vi "Handshake.vi"(8 "error in (no error)":errorcluster, 9 "Timeout (5000ms)":i32=5000, 11 "dotNET SSL Socket in":refnum<class "dotNET SSL Server.lvclass">) -> (0 "error out":errorcluster, 3 "dotNET SSL Socket out":refnum<class "dotNET SSL Server.lvclass">)   [LabVIEW 2013, in "dotNET SSL Socket.lvlib" / "dotNET SSL Server.lvclass"]
doc: "Performs the SSL Server handshake."
uses:
  dotNET SSL Server.lvclass
  dotNET SSL Socket/dotNET SSL Socket.lvclass/dotNET SSL Socket.ctl
  dotNET SSL Server.lvclass/dotNET SSL Server.ctl
  dotNET SSL Socket/Read SSLStream.vi
  Read Client Cert Required.vi
  dotNET SSL Socket/Read Check Revocation.vi
  Read Server Certificate.vi
  dotNET SSL Socket/Read Masked SSL Protocols.vi
  dotNET SSL Socket/dotNET SSL Socket.lvclass
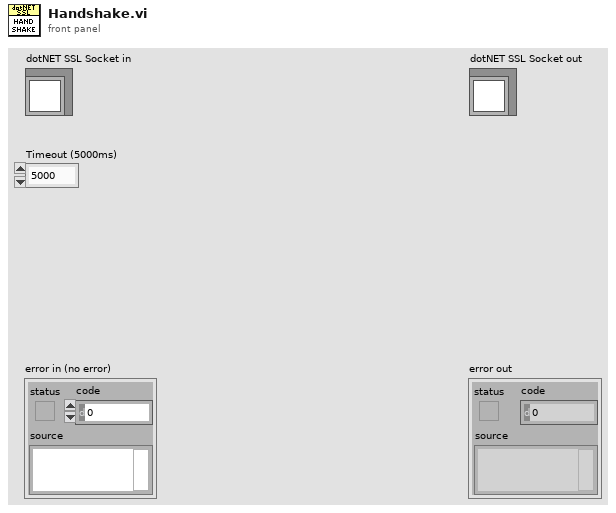
[diagram p1: front panel]
types:
  T1 = typedef "dotNET SSL Socket.lvlib/dotNET SSL Socket.lvclass/PFX Certificate.ctl" = cluster{"PFX Certificate":path, "PFX Password":string}
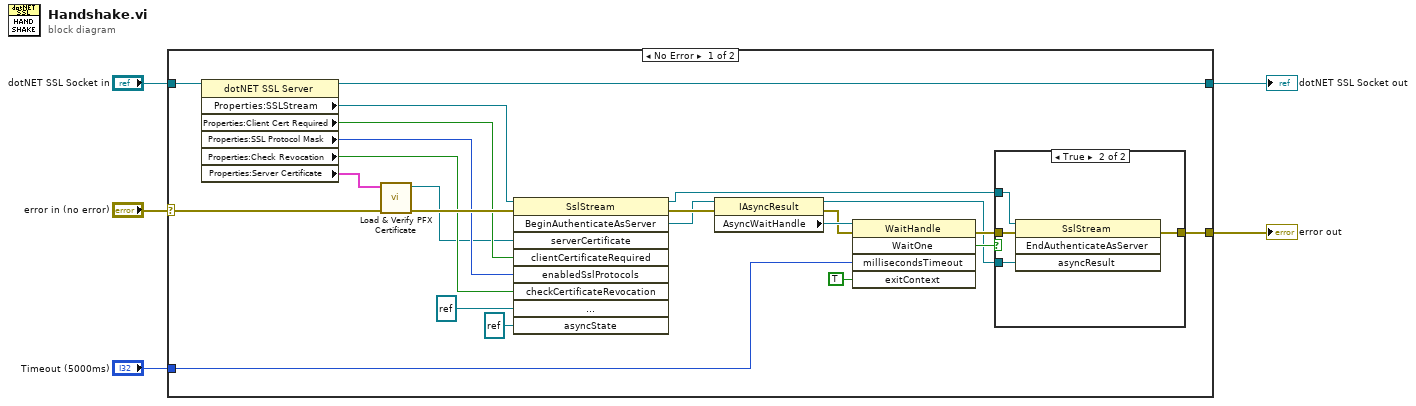
[diagram p0: block diagram]
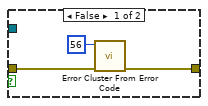
[diagram p2: hidden frame]
diagram:
  n1 = case shown="No Error" "error in (no error)" {
    selector: "error in (no error)" -> [w28 w37]
    tunnel: [w15 w37] -> w4
    tunnel: [w24 w36] -> w2
    tunnel: "dotNET SSL Socket in" -> [w26 w36]
    tunnel: "Timeout (5000ms)" -> [w19 _]
    frame No Error {
      n2 = property class="dotNET SSL Server"(reference=w26) -> (reference out=w24:refnum<class "dotNET SSL Server.lvclass">, "Properties:SSLStream"=w25:refnum<k24>, "Properties:Client Cert Required"=w12:bool, "Properties:SSL Protocol Mask"=w8:i32, "Properties:Check Revocation"=w9:bool, "Properties:Server Certificate"=w6:T1)  [unwired: 1 in, 1 out]
      n3 = call "Load & Verify PFX Certificate.vi"("error in (no error)"=w28, "PFX Certificate in"=w6) -> ("error out"=w27:errorcluster, "X509 Certificate out"=w7:refnum<k24>)  [unwired: 8 in]
      n4 = invoke class="SslStream" method="BeginAuthenticateAsServer"(reference=w25, error in=w27, "serverCertificate"=w7, "clientCertificateRequired"=w12, "enabledSslProtocols"=w8, "checkCertificateRevocation"=w9, "asyncCallback"=refnum<k24> refnum, "asyncState"=refnum<k24> refnum) -> (reference out=w13:refnum<k24>, error out=w23:errorcluster, "BeginAuthenticateAsServer"=w22:refnum<k24>)  [unwired: 1 in, 6 out]
      n5 = property class="IAsyncResult"(reference=w22, error in=w23) -> (reference out=w14:refnum<k24>, error out=w20:errorcluster, "AsyncWaitHandle"=w21:refnum<k24>)
      n6 = invoke class="WaitHandle" method="WaitOne"(reference=w21, error in=w20, "millisecondsTimeout"=w19, "exitContext"=TRUE) -> (error out=w16:errorcluster, "WaitOne"=w17:bool)  [unwired: 1 in, 3 out]
      n7 = case shown="True" w17 {
        tunnel: w16 -> [w30 w35]
        tunnel: [w29 w33] -> w15
        tunnel: w14 -> [_ w34]
        tunnel: w13 -> [_ w32]
        frame False {
          n8 = call <vilib>:"Error Cluster From Error Code.vi"("error in (no error)"=w30, "error code (0)"=56) -> ("error out"=w29:errorcluster)  [unwired: 7 in]
        }
        frame True {
          n9 = invoke class="SslStream" method="EndAuthenticateAsServer"(reference=w32, error in=w35, "asyncResult"=w34) -> (error out=w33:errorcluster)  [unwired: 1 in, 3 out]
        }
      }
    }
    frame Error {
    }
  }
  "error out" <- w4
  "dotNET SSL Socket out" <- w2
